vi "Robot Controller 1.vi"() -> ()   [LabVIEW 2014]
panel:
  in  "Tab Control":T1(tab)
  out "Heading":dbl(knob) scale=0.0..360.0
  in  "Steer Angle":dbl(knob) scale=0.0..360.0
  out "Commanded Steering Angle":dbl(graph)
  in  "Steering Angle Debug":dbl(knob) scale=0.0..360.0
  out "Desired & Measured Headings":cluster{"Desired Heading":dbl, dbl}(graph)
  in  "Desired Heading":dbl(slide) scale=0.0..360.0
  in  "Emergency Stop":bool
  out "Robot Active":bool
  # "To run press arrow above"
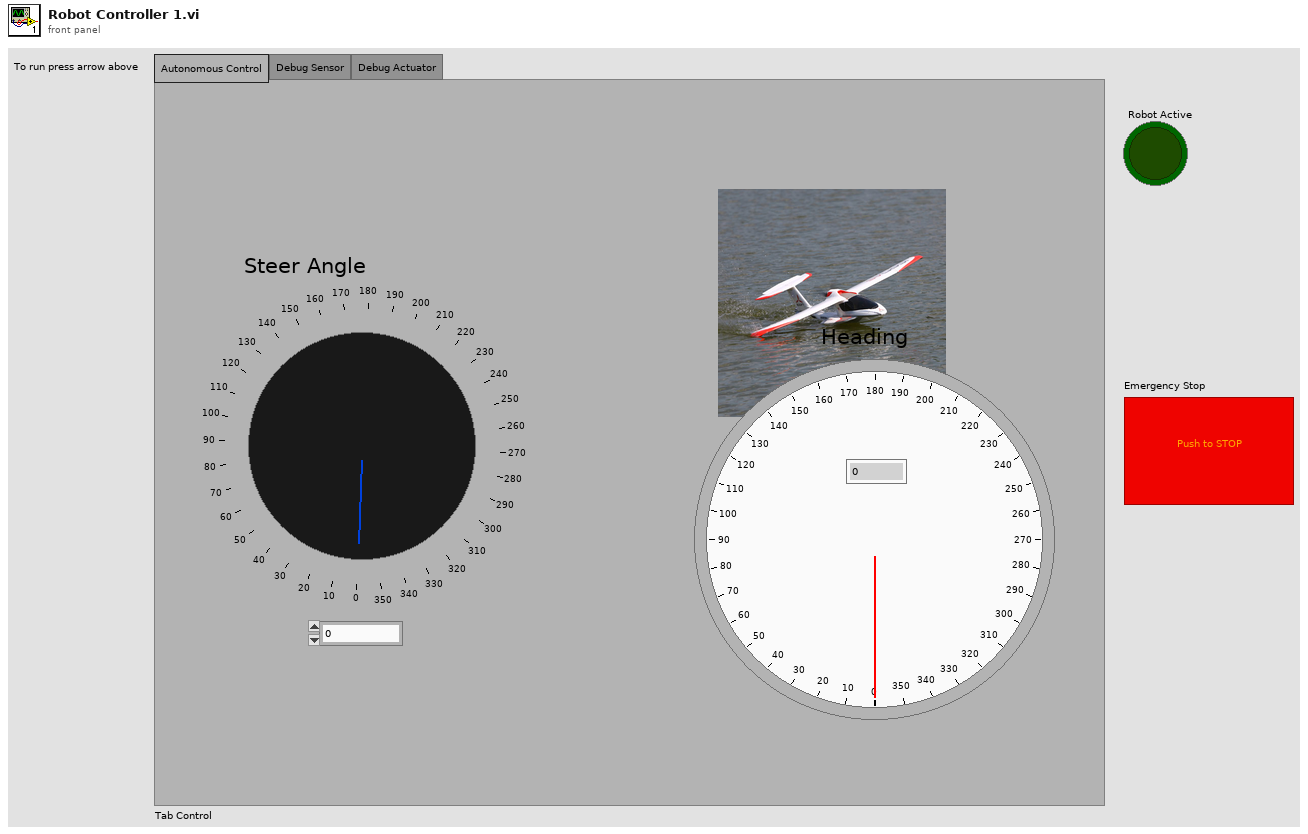
[diagram p1: front panel]
types:
  T1 = enum32{"Autonomous Control", "Debug Sensor", "Debug Actuator"}
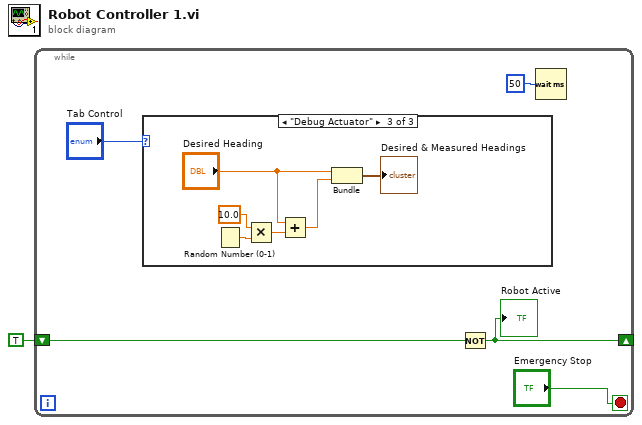
[diagram p0: block diagram]
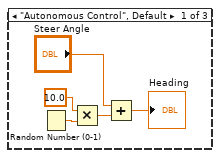
[diagram p2: hidden frame]
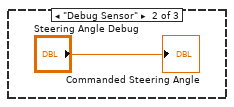
[diagram p3: hidden frame]
diagram:
  n1 = while {
    shift-right: [w4] -> _
    shift-left: TRUE -> [w6]
    stop <- "Emergency Stop" stop-if-true
    n2 = case shown="\"Debug Actuator\"" "Tab Control" {
      frame "Autonomous Control", Default {
        n3 = Random Number (0-1)() -> (number: 0 to 1=w7:dbl)
        n4 = Multiply(x=10.0, y=w7) -> (x*y=w9:dbl)
        n5 = Add(x="Steer Angle", y=w9) -> (x+y=→"Heading":dbl)
      }
      frame "Debug Sensor" {
        "Commanded Steering Angle" <- "Steering Angle Debug"
      }
      frame "Debug Actuator" {
        n6 = Random Number (0-1)() -> (number: 0 to 1=w17:dbl)
        n7 = Multiply(x=10.0, y=w17) -> (x*y=w15:dbl)
        n8 = Add(x="Desired Heading", y=w15) -> (x+y=w13:dbl)
        n9 = Bundle("Desired Heading"="Desired Heading", w13) -> (→"Desired & Measured Headings":cluster{"Desired Heading":dbl, dbl})  [unwired: 1 in]
      }
    }
    n10 = Not(x=w6) -> (.not. x?=w4:bool)
    "Robot Active" <- w4
    n11 = Wait (ms)(milliseconds to wait=u32 50) -> ()  [unwired: 1 out]
  }
